vi "Add Label.vi"(8 "error in":errorcluster, 10 "label":T2, 11 "port ref":T1 format="%.0x") -> (0 "error out":errorcluster, 3 "port ref out":T1 format="%.0x")   [LabVIEW 2020, in "Ballard ARINC 429 Scripting.lvlib"]
uses:
  Ballard ARINC 429 Scripting.lvlib
  Shared/Label Properties.ctl
  <vilib>/NI VeriStand/Custom Device API/Custom Device API.lvlib
  Constants.vi
  <vilib>/NI VeriStand/Custom Device API/Custom Device Item Ref.ctl
  Encoding and Decoding/Encoding.ctl
  Encoding and Decoding/Encoding and Decoding.lvlib
  Shared/Parameter Definition.ctl
  Shared/Direction.ctl
  Shared/VS Channel Definition for Parameter.ctl
  Shared/VS Channels Definition for Label.ctl
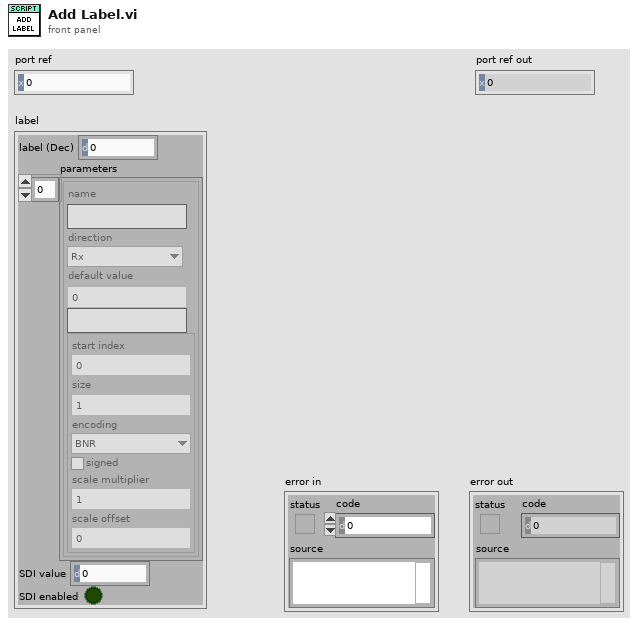
[diagram p1: front panel]
types:
  T1 = typedef "Custom Device API.lvlib/Custom Device Item Ref.ctl" = u64
  T2 = typedef "VS Channels Definition for Label.ctl" = cluster{"label (Dec)":i32, "parameters":T3[], "SDI value":u8, "SDI enabled":bool}
  T3 = typedef "VS Channel Definition for Parameter.ctl" = cluster{"name":string, "direction":T4, "default value":dbl, "unit":string, "Parameter":T5}
  T4 = typedef "Direction.ctl" = enum16{"Rx", "Tx"}
  T5 = typedef "Parameter Definition.ctl" = cluster{"start index":i32, "size":i32, "encoding":T6, "signed":bool, "scale multiplier":dbl, "scale offset":dbl}
  T6 = typedef "Encoding and Decoding.lvlib/Encoding.ctl" = enum16{"BNR", "BCD", "Discrete"}
  T7 = typedef "Label Properties.ctl" = cluster{"label (Dec)":i32, "SDI value":u8, "SDI enabled":bool}
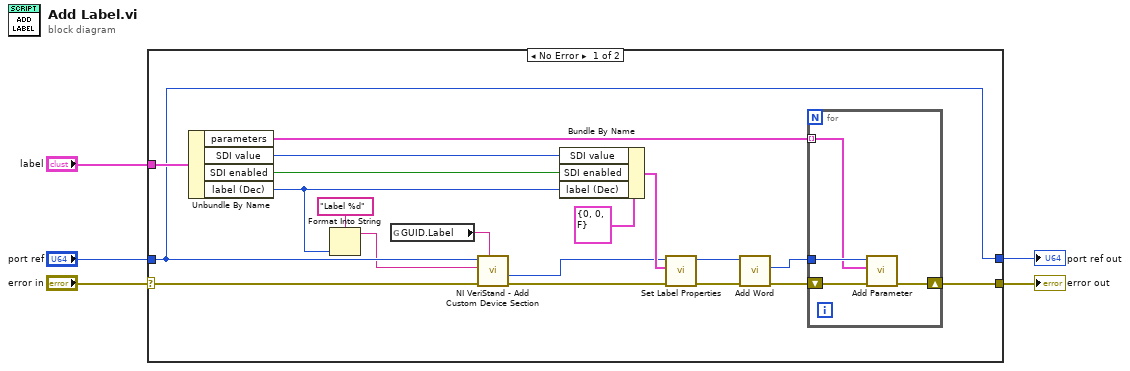
[diagram p0: block diagram]
diagram:
  n1 = case shown="No Error" "error in" {
    selector: "error in" -> [w24 w30]
    tunnel: "port ref" -> [w21 w29]
    tunnel: [w23 w30] -> w4
    tunnel: "label" -> [w22 _]
    tunnel: [w21 w29] -> w1
    frame No Error {
      n2 = Unbundle By Name(w22) -> ("parameters"=w6:T3[], "SDI value"=w15:u8, "SDI enabled"=w16:bool, "label (Dec)"=w17:i32)
      n3 = Format Into String(format string="Label %d", w17) -> (resulting string=w8:string)  [unwired: 2 in, 1 out]
      n4 = global read "Constants.vi" "GUID.Label"() -> (w7:string)
      n5 = call <vilib>:"NI VeriStand - Add Custom Device Section.vi"("GUID (Default Section)"=w7, "error in (no error)"=w24, "Section Name"=w8, "Parent Ref in"=w21) -> ("error out"=w10:errorcluster, "Section Ptr"=w9:T1)  [unwired: 4 in, 2 out]
      n6 = Bundle By Name(cluster=T7 {"label (Dec)"=0, "SDI value"=0, "SDI enabled"=FALSE} ("label properties"), "SDI value"=w15, "SDI enabled"=w16, "label (Dec)"=w17) -> (w19:T7)
      n7 = call "Set Label Properties.vi"("error in"=w10, "label properties"=w19, "label ref"=w9) -> ("error out"=w14:errorcluster, "label ref out"=w12:T1)  [unwired: 7 in]
      n8 = call "Add Word.vi"("error in"=w14, "label ref"=w12) -> ("error out"=w13:errorcluster, "word ref"=w11:T1)  [unwired: 6 in, 2 out]
      n9 = for {
        shift-right: [w26] -> w23
        shift-left: w13 -> [w27]
        tunnel: w6 -> [w25] mode=indexing
        tunnel: w11 -> [w28]
        n10 = call "Add Parameter.vi"("error in"=w27, "parameter"=w25, "word ref"=w28) -> ("error out"=w26:errorcluster)  [unwired: 6 in, 2 out]
      }
    }
    frame Error {
    }
  }
  "error out" <- w4
  "port ref out" <- w1
